vi "Set Sessions_ksENA.vi"(11 "Semiconductor Module Context":T1) -> (0 "error out":errorcluster)   [LabVIEW 2013]
uses:
  <vilib>/NI_TestStand_SemiconductorModule/NI_TestStand_Semiconductor_Module.lvlibp/PinMap/General/SemiconductorModuleContext.ctl
  <vilib>/NI_TestStand_SemiconductorModule/NI_TestStand_Semiconductor_Module.lvlibp
  DMM/Pin Map API/DMM Custom Instruments.lvlib
  ENA/Pin Map API/ENA Custom Instrument.lvlib
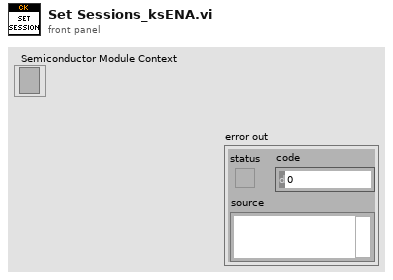
[diagram p1: front panel]
types:
  T1 = typedef "NI_TestStand_Semiconductor_Module.lvlibp/SemiconductorModuleContext.ctl" = refnum<k7>
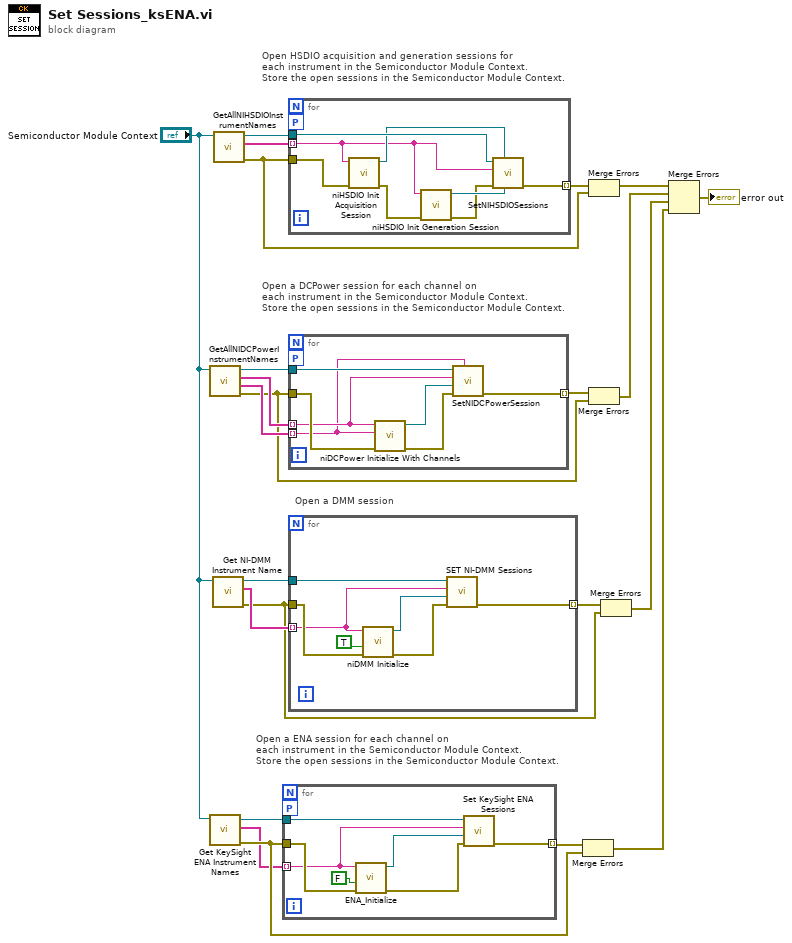
[diagram p0: block diagram]
diagram:
  # "Open a ENA session for each channel on \neach instrument in the Semiconductor Module Context.\nStore the open sessions in the Semiconductor Module Context."
  # "Open a DMM session"
  # "Open a DCPower session for each channel on \neach instrument in the Semiconductor Module Context.\nStore the open sessions in the Semiconductor Module Context."
  # "Open HSDIO acquisition and generation sessions for\neach instrument in the Semiconductor Module Context.\nStore the open sessions in the Semiconductor Module Context."
  n1 = call <vilib>:"GetAllNIDCPowerInstrumentNames.vi"("Semiconductor Module Context"="Semiconductor Module Context") -> ("error out"=w15:errorcluster, "Channel Ids"=w19:string[], "Instrument Names"=w22:string[], "Semiconductor Module Context Out"=w21:T1)  [unwired: 7 in]
  n2 = call "Get KeySight ENA Instrument Names.vi"("Semiconductor Module Context"="Semiconductor Module Context") -> ("error out"=w5:errorcluster, "Instrument Names"=w3:string[], "Semiconductor Module Context Out"=w4:T1)  [unwired: 7 in, 1 out]
  n3 = call "Get NI-DMM Instrument Name.vi"("Semiconductor Module Context"="Semiconductor Module Context") -> ("Semiconductor Module Context Out"=w11:T1, "Instrument Names"=w10:string[], "error out"=w8:errorcluster)  [unwired: 6 in, 1 out]
  n4 = call <vilib>:"GetAllNIHSDIOInstrumentNames.vi"("Semiconductor Module Context"="Semiconductor Module Context") -> ("error out"=w12:errorcluster, "Instrument Names"=w23:string[], "Semiconductor Module Context Out"=w18:T1)  [unwired: 8 in]
  n5 = for {
    tunnel: w3 -> [w25] mode=indexing
    workers-P: _ -> [_]
    tunnel: w5 -> [w26]
    tunnel: [w30] -> w6 mode=indexing
    tunnel: w4 -> [w29]
    n6 = call "ENA_Initialize.vi"("error in (no error)"=w26, "Reset? (T: Yes)"=FALSE, "VISA resource name"=w25) -> ("error out"=w27:errorcluster, "VISA resource name out"=w24:refnum<visa-resource-name>)  [unwired: 7 in]
    n7 = call "Set KeySight ENA Sessions.vi"("error in (no error)"=w27, "Instrument Session"=w24, "Instrument Name"=w25, "Semiconductor Module Context"=w29) -> ("error out"=w30:errorcluster)  [unwired: 6 in, 1 out]
  }
  n8 = for {
    tunnel: w23 -> [w32] mode=indexing
    tunnel: w12 -> [w38]
    tunnel: [w34] -> w13 mode=indexing
    tunnel: w18 -> [w37]
    workers-P: _ -> [_]
    n9 = call <instrlib>:"niHSDIO Init Acquisition Session.vi"("error in (no error)"=w38, "resource name"=w32) -> ("error out"=w33:errorcluster, "instrument handle out"=w36:refnum<k15>)  [unwired: 8 in]
    n10 = call <instrlib>:"niHSDIO Init Generation Session.vi"("error in (no error)"=w33, "resource name"=w32) -> ("error out"=w31:errorcluster, "instrument handle out"=w35:refnum<k15>)  [unwired: 8 in]
    n11 = call <vilib>:"SetNIHSDIOSessions.vi"("Generation Session"=w35, "Acquisition Session"=w36, "error in (no error)"=w31, "Instrument Name"=w32, "Semiconductor Module Context"=w37) -> ("error out"=w34:errorcluster)  [unwired: 5 in, 1 out]
  }
  n12 = for {
    tunnel: w22 -> [w42] mode=indexing
    tunnel: w19 -> [w39] mode=indexing
    workers-P: _ -> [_]
    tunnel: w15 -> [w43]
    tunnel: [w44] -> w17 mode=indexing
    tunnel: w21 -> [w45]
    n13 = call <instrlib>:"niDCPower Initialize With Channels.vi"("error in (no error)"=w43, "channels"=w39, "resource name"=w42) -> ("error out"=w41:errorcluster, "instrument handle out"=w40:refnum<k15>)  [unwired: 7 in]
    n14 = call <vilib>:"SetNIDCPowerSession.vi"("Channel Id"=w39, "error in (no error)"=w41, "Instrument Session"=w40, "Instrument Name"=w42, "Semiconductor Module Context"=w45) -> ("error out"=w44:errorcluster)  [unwired: 5 in, 1 out]
  }
  n15 = for {
    tunnel: w10 -> [w48] mode=indexing
    tunnel: w11 -> [w50]
    tunnel: w8 -> [w52]
    tunnel: [w49] -> w9 mode=indexing
    n16 = call <instrlib>:"niDMM Initialize.vi"("error in (no error)"=w52, "Reset"=TRUE ("ID Query"), "Instrument Descriptor"=w48) -> ("error out"=w51:errorcluster, "instrument handle out"=w47:refnum<k15>)  [unwired: 7 in]
    n17 = call "SET NI-DMM Sessions.vi"("error in (no error)"=w51, "Instrument Session"=w47, "Instrument Name"=w48, "Semiconductor Module Context"=w50) -> ("error out"=w49:errorcluster)  [unwired: 6 in, 1 out]
  }
  n18 = Merge Errors(w6, w5) -> (w1:errorcluster)
  n19 = Merge Errors(w13, w12) -> (w14:errorcluster)
  n20 = Merge Errors(w17, w15) -> (w16:errorcluster)
  n21 = Merge Errors(w9, w8) -> (w7:errorcluster)
  n22 = Merge Errors(w14, w16, w7, w1) -> (→"error out":errorcluster)
